vi "Read Publisher ID.vi"(11 "PublishRequest In":refnum<class "PublishRequest.lvclass">) -> (2 "Publisher ID":string)   [LabVIEW 2017, in "IMediator.lvlib" / "PublishRequest.lvclass"]
uses:
  PublishRequest.lvclass
  PublishRequest.lvclass/PublishRequest.ctl
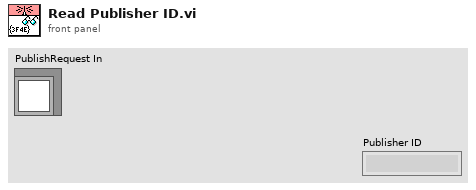
[diagram p1: front panel]
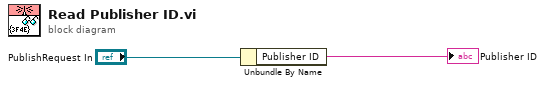
[diagram p0: block diagram]
diagram:
  n1 = Unbundle By Name("PublishRequest In") -> ("Publisher ID"=→"Publisher ID":string)
